vi "Choose Random Value from Preferred Array.vi"(0 "Preferred Array":i32[](array[numeric]), 5 "Backup Array":i32[](array[numeric])) -> (2 "Array Out":i32[](array[numeric]), 3 "Empty Array?":bool, 4 "Selected Value":i32, 6 "Selected Index":i32)   [LabVIEW 2014]
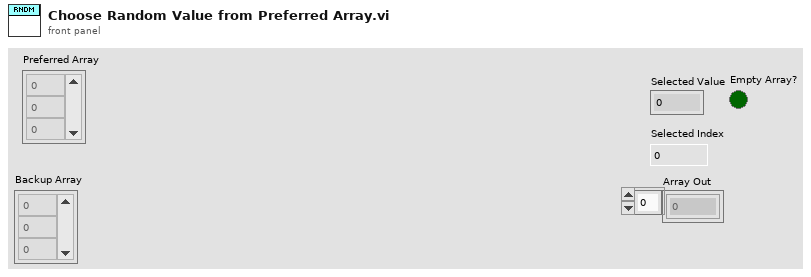
[diagram p1: front panel]
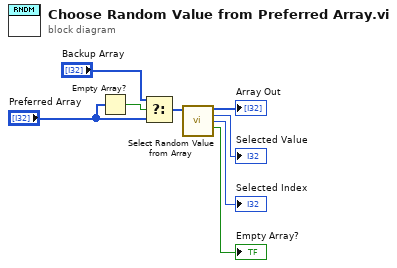
[diagram p0: block diagram]
diagram:
  n1 = Empty Array?(array="Preferred Array") -> (empty?=w6:bool)
  n2 = Select(t="Backup Array", s=w6, f="Preferred Array") -> (s? t:f=w5:i32[])
  n3 = call "Select Random Value from Array.vi"("Array"=w5) -> ("Array Out"=→"Array Out":i32[], "Selected Value"=→"Selected Value":i32, "Selected Index"=→"Selected Index":i32, "Empty Array?"=→"Empty Array?":bool)  [unwired: 11 in]
